vi "Get_File_Info_Listing.vi"(0 "path":path) -> (1 "Path":path[](array[path]), 2 "Last Mod":timestamp[](array[timestamp]), 3 "Size":i64[](array[numeric]))   [LabVIEW 2011]
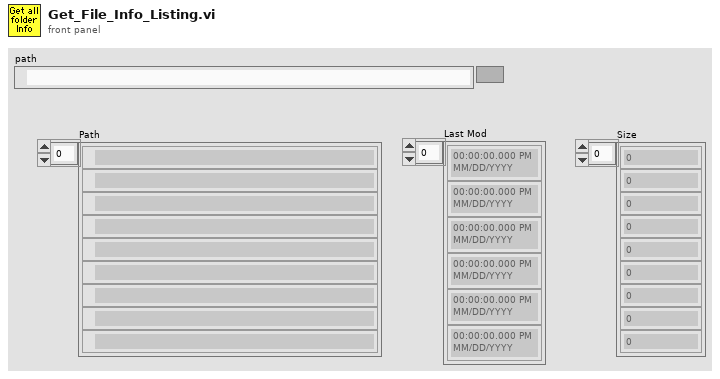
[diagram p1: front panel]
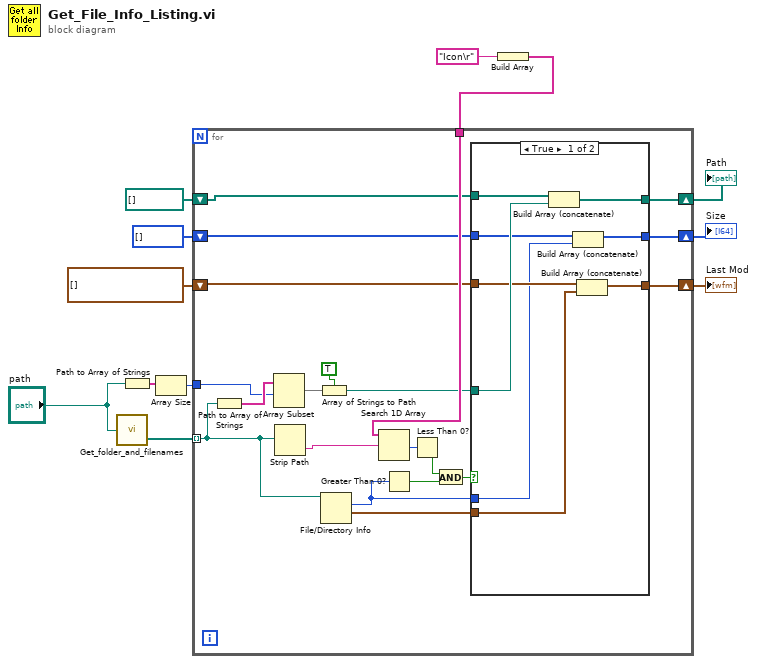
[diagram p0: block diagram]
diagram:
  n1 = call "Get_folder_and_filenames.vi"("file path (dialog if empty)"="path") -> ("Files"=w8:path[])  [unwired: 1 out]
  n2 = Path to Array of Strings(0:"path") -> (2:w9:string[])  [unwired: 1 out]
  n3 = Array Size(array=w9) -> (size(s)=w10:i32)
  n4 = Build Array("Icon\r") -> (w12:string[])
  n5 = for {
    tunnel: w8 -> [w18] mode=indexing
    tunnel: w10 -> [w31]
    shift-right: [w23] -> w1
    shift-left: path[] [] -> [w25]
    tunnel: w12 -> [w29]
    shift-right: [w21] -> w2
    shift-left: i64[] [] -> [w22]
    shift-right: [w19] -> w3
    shift-left: timestamp[] [] -> [w20]
    n6 = Path to Array of Strings(0:w18) -> (2:w32:string[])  [unwired: 1 out]
    n7 = Array Subset(array=w32, index=w31) -> (w27:string[])  [unwired: 1 in]
    n8 = Strip Path(path=w18) -> (name=w30:string)  [unwired: 1 out]
    n9 = Array of Strings to Path(0:w27, 1:TRUE ("relative")) -> (2:w24:path)
    n10 = File/Directory Info(path=w18) -> (size=w13:i64, last mod=w14:timestamp)  [unwired: 1 in, 5 out]
    n11 = Search 1D Array(1D array=w29, element=w30) -> (index of element=w28:i32)  [unwired: 1 out]
    n12 = Greater Than 0?(x=w13) -> (x > 0?=w16:bool)
    n13 = Less Than 0?(x=w28) -> (x < 0?=w17:bool)
    n14 = And(x=w17, y=w16) -> (x .and. y?=w15:bool)
    n15 = case shown="True" w15 {
      tunnel: w25 -> [w41 w44]
      tunnel: w24 -> [w40 _]
      tunnel: [w39 w44] -> w23
      tunnel: w22 -> [w38 w43]
      tunnel: [w37 w43] -> w21
      tunnel: w20 -> [w36 w42]
      tunnel: [w35 w42] -> w19
      tunnel: w14 -> [w34 _]
      tunnel: w13 -> [w33 _]
      frame True {
        n16 = Build Array (concatenate)(w41, w40) -> (w39:path[])
        n17 = Build Array (concatenate)(w38, w33) -> (w37:i64[])
        n18 = Build Array (concatenate)(w36, w34) -> (w35:timestamp[])
      }
      frame False {
      }
    }
  }
  "Last Mod" <- w3
  "Size" <- w2
  "Path" <- w1
